vi "Stop Object.vi"(8 "error in (no error)":errorcluster, 10 "Name":string, 11 "Da Base in":refnum<class "Template Module.lvclass">) -> (0 "error out":errorcluster, 3 "Da Base out":refnum<class "Template Module.lvclass">)   [LabVIEW 2019, in "Template Module.lvclass"]
uses:
  Template Module.lvclass
  Template Module.lvclass/Template Module.ctl
  <vilib>/ActorFramework/Message Enqueuer/Message Enqueuer.lvclass/Message Enqueuer.ctl
  <vilib>/ActorFramework/Message Enqueuer/Enqueue.vi
  <vilib>/ActorFramework/Stop Msg/Stop Msg.lvclass
  C:/Program Files/National Instruments/LabVIEW 2019/vi.lib/ActorFramework/Message/Message.lvclass
  <vilib>/ActorFramework/Message Priority Queue/Priority Enqueue.vi
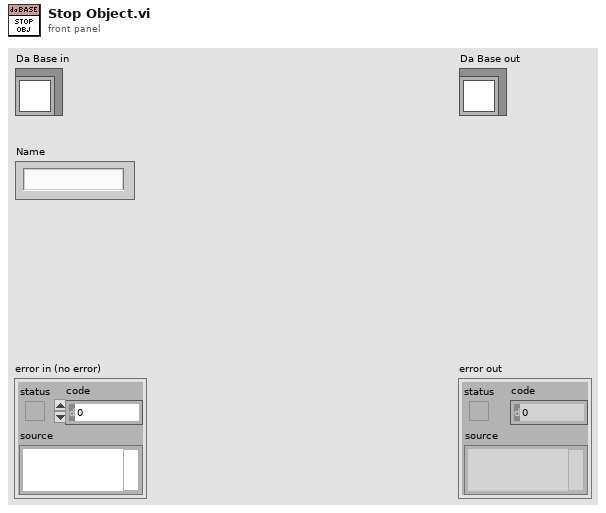
[diagram p1: front panel]
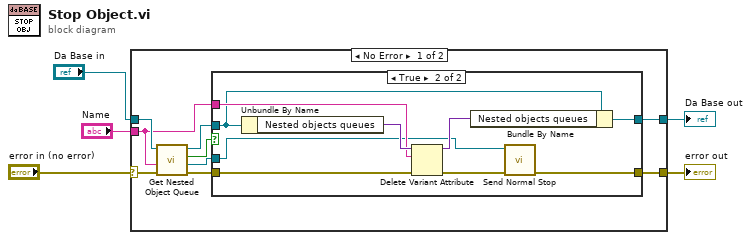
[diagram p0: block diagram]
diagram:
  n1 = case shown="No Error" "error in (no error)" {
    selector: "error in (no error)" -> [w7 w27]
    tunnel: [w6 w27] -> w4
    tunnel: [w9 w26] -> w2
    tunnel: "Da Base in" -> [w14 w26]
    tunnel: "Name" -> [w11 _]
    frame No Error {
      n2 = call-dynamic "Get Nested Object Queue.vi"("error in (no error)"=w7, "Name"=w11, "Measure Object in"=w14) -> ("error out"=w10:errorcluster, "Object Enqueuer"=w8:refnum<class "Message Enqueuer.lvclass">, "Found?"=w13:bool, "Measure Object out"=w12:refnum<class "Template Module.lvclass">)  [unwired: 5 in]
      n3 = case shown="True" w13 {
        tunnel: w12 -> [w16 w22]
        tunnel: w11 -> [_ w24]
        tunnel: w10 -> [w15 w23]
        tunnel: [w16 w19] -> w9
        tunnel: w8 -> [_ w18]
        tunnel: [w15 w17] -> w6
        frame False {
        }
        frame True {
          n4 = Unbundle By Name(w22) -> ("Nested objects queues"=w25:variant)
          n5 = Delete Variant Attribute(4:w23, 6:w24, 7:w25) -> (0:w20:errorcluster, 3:w21:variant)  [unwired: 1 out]
          n6 = Bundle By Name(cluster=w22, "Nested objects queues"=w21) -> (w19:refnum<class "Template Module.lvclass">)
          n7 = call <vilib>:"Send Normal Stop.vi"("error in (no error)"=w20, "Message Enqueuer"=w18) -> ("error out"=w17:errorcluster)  [unwired: 9 in]
        }
      }
    }
    frame Error {
    }
  }
  "error out" <- w4
  "Da Base out" <- w2
